vi "SS2 Live_Close Communication.vi"(8 "Error In":errorcluster, 10 "Device Refnum":refnum<k24>, 11 "okCFrontPanelDevices Refnum":refnum<k24>) -> (0 "Error Out":errorcluster)   [LabVIEW 2019]
uses:
  C:/UCLA Thinkpad Google Drive/LabVIEW 2019 SP1/builds/SS2 Live Distribution/Opal Kelly/C# Wrapper/libFrontPanel-csharp.dll
  Opal Kelly/C# Wrapper/libFrontPanel-csharp.dll
  Opal Kelly/C# Wrapper/okFrontPanelC#Wrapper.lvlib
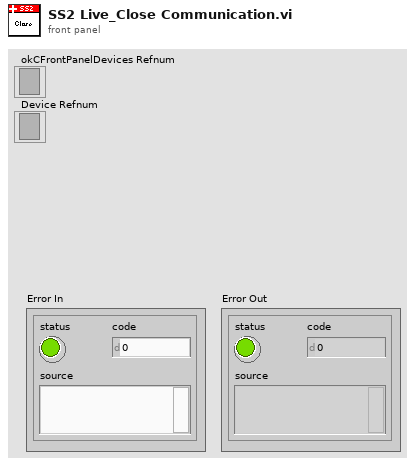
[diagram p1: front panel]
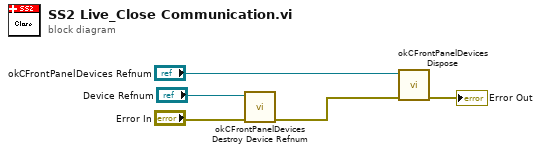
[diagram p0: block diagram]
diagram:
  n1 = call "okCFrontPanelDevices Destroy Device Refnum.vi"("error in (no error)"="Error In", "okCFrontPanel Device Refnum"="Device Refnum") -> ("error out"=w3:errorcluster)  [unwired: 9 in]
  n2 = call "okCFrontPanelDevices Dispose.vi"("Error In"=w3, "okCFrontPanelDevices Refnum"="okCFrontPanelDevices Refnum") -> ("Error Out"=→"Error Out":errorcluster)  [unwired: 9 in]
